vi "RT_Angle_Of_Attack_in_DLR_Navigation_Reference_System (SubVI).vi"(9 "V_wind (m/s)":dbl[](array[numeric]), 10 "V (m/s)":dbl[](array[numeric]), 11 "DCM":dbl[][](array[numeric])) -> (2 "AoA_yaw (rad)":dbl, 3 "AoA_pitch (rad)":dbl)   [LabVIEW 2017]
uses:
  <vilib>/Analysis/Matrix/Datatypes/RealMatrix.ctl
  <vilib>/Analysis/baseanly.llb/Real A x B.vi
  <vilib>/Analysis/Matrix/Numeric/Conversions/Array To Matrix - RA2.vi
  <vilib>/Analysis/Matrix/Numeric/Conversions/Matrix To Array - RM.vi
  <vilib>/Analysis/NI_AALBase.lvlib
  <vilib>/Analysis/Matrix/NI_Matrix.lvlib
panel:
  out "r":dbl[](array[numeric])
  out "v":dbl[](array[numeric])
  out "r_matrix":T1
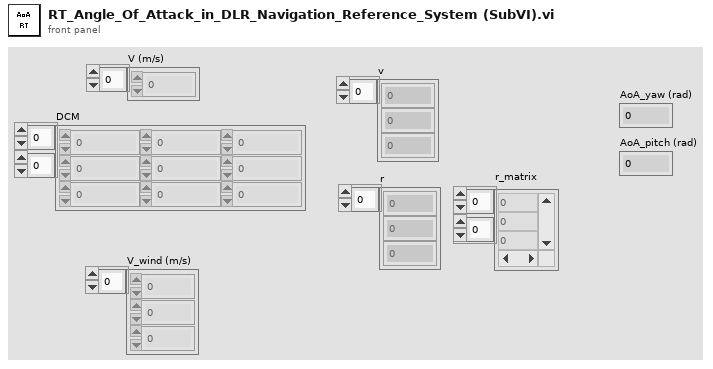
[diagram p1: front panel]
types:
  T1 = typedef "NI_Matrix.lvlib/RealMatrix.ctl" = dbl[][]
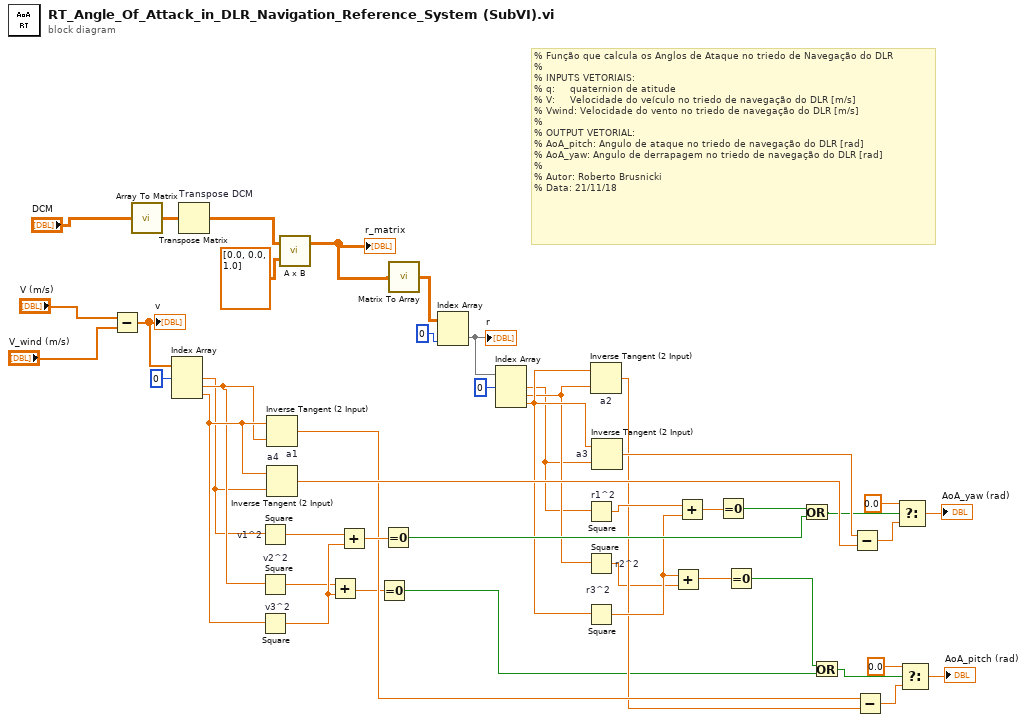
[diagram p0: block diagram]
diagram:
  # "% Função que calcula os Anglos de Ataque no triedo de Navegação do DLR \n%\n% INPUTS VETORIAIS: \n% q:     quaternion de atitude   \n% V:     Velocidade do veículo no triedo de navegação do DLR [m/s]\n% Vwind: Velocidade do vento no triedo de navegação do DLR [m/s]\n%\n% OUTPUT VETORIAL:\n% AoA_pitch: Angulo de ataque no triedo de navegação do DLR [rad]\n% AoA_yaw: Angulo de derrapagem no triedo de navegação do DLR [rad]\n%\n% Autor: Roberto Brusnicki\n% Data: 21/11/18"
  n1 = Subtract(x="V (m/s)", y="V_wind (m/s)") -> (x-y=w13:dbl[])
  "v" <- w13
  n2 = call-poly <vilib>:"Array To Matrix.vi"("Real 2D Array"="DCM") -> ("Real Matrix"=w5:T1)
  n3 = Index Array(array=w13, index #1=0 ("index (row)")) -> (element #1=w14:dbl, element #2=w15:dbl, element #3=w16:dbl)  [unwired: 2 in]
  n4 = Transpose Matrix "Transpose DCM"(1:w5) -> (0:w6:T1)
  n5 = Square "v1^2"(x=w14) -> (x^2=w32:dbl)
  n6 = Square "v2^2"(x=w15) -> (x^2=w20:dbl)
  n7 = Square "v3^2"(x=w16) -> (x^2=w33:dbl)
  n8 = Inverse Tangent (2 Input) "a1"(1:w15, 2:w16) -> (0:w29:dbl)
  n9 = Inverse Tangent (2 Input) "a4"(1:w14, 2:w16) -> (0:w44:dbl)
  n10 = call-poly <vilib>:"A x B.vi"("B"=T1 [[0.0], [0.0], [1.0]], "A"=w6) -> ("A x B"=w3:T1)  [unwired: 1 out]
  "r_matrix" <- w3
  n11 = Add(x=w20, y=w33) -> (x+y=w23:dbl)
  n12 = Add(x=w32, y=w33) -> (x+y=w34:dbl)
  n13 = Equal To 0?(x=w23) -> (x = 0?=w25:bool)
  n14 = Equal To 0?(x=w34) -> (x = 0?=w38:bool)
  n15 = call-poly <vilib>:"Matrix To Array.vi"("Real Matrix"=w3) -> ("Real 2D Array"=w9:dbl[][])
  n16 = Index Array(array=w9, index (col)=0 ("index (row)")) -> (element=w11:dbl[])  [unwired: 1 in]
  "r" <- w11
  n17 = Index Array(array=w11, index #1=0 ("index (row)")) -> (element #1=w17:dbl, element #2=w18:dbl, element #3=w19:dbl)  [unwired: 2 in]
  n18 = Square "r1^2"(x=w17) -> (x^2=w35:dbl)
  n19 = Square "r2^2"(x=w18) -> (x^2=w21:dbl)
  n20 = Square "r3^2"(x=w19) -> (x^2=w36:dbl)
  n21 = Inverse Tangent (2 Input) "a2"(1:w18, 2:w19) -> (0:w28:dbl)
  n22 = Inverse Tangent (2 Input) "a3"(1:w17, 2:w19) -> (0:w45:dbl)
  n23 = Add(x=w36, y=w21) -> (x+y=w22:dbl)
  n24 = Add(x=w35, y=w36) -> (x+y=w37:dbl)
  n25 = Equal To 0?(x=w37) -> (x = 0?=w39:bool)
  n26 = Equal To 0?(x=w22) -> (x = 0?=w24:bool)
  n27 = Or(x=w39, y=w38) -> (x .or. y?=w43:bool)
  n28 = Or(x=w24, y=w25) -> (x .or. y?=w26:bool)
  n29 = Subtract(x=w45, y=w44) -> (x-y=w41:dbl)
  n30 = Subtract(x=w29, y=w28) -> (x-y=w30:dbl)
  n31 = Select(t=0.0, s=w43, f=w41) -> (s? t:f=→"AoA_yaw (rad)":dbl)
  n32 = Select(t=0.0, s=w26, f=w30) -> (s? t:f=→"AoA_pitch (rad)":dbl)
